vi "Flash LED.vi"(8 "Error In":errorcluster, 10 "Interval (S) (1 S)":dbl=1.0) -> (0 "Error Out":errorcluster, 2 "LED State":bool)   [LabVIEW 2016]
doc: "Toggles the USER LED on the cRIO at the specified when repetitively called.\nIt is designed to show genuine activity and will not cause the LED to Flash unless repetitively called\nat an interval shorter than the Interval. DR 11-10-2011"
uses:
  <vilib>/NI_Real-Time Target Support.lvlib
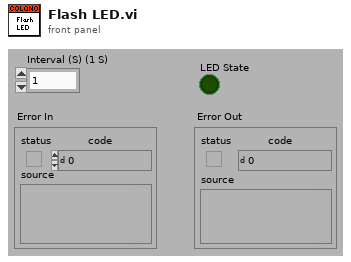
[diagram p1: front panel]
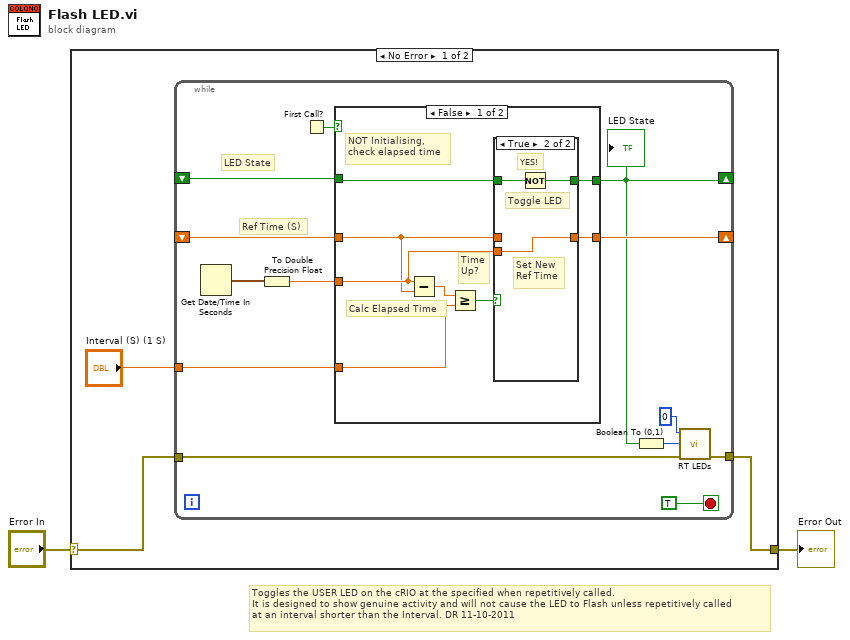
[diagram p0: block diagram]
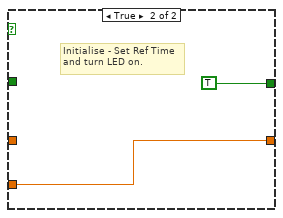
[diagram p3: hidden frame]
diagram:
  # "Toggles the USER LED on the cRIO at the specified when repetitively called.\nIt is designed to show genuine activity and will not cause the LED to Flash unless repetitively called\nat an interval shorter than the Interval. DR 11-10-2011"
  n1 = case shown="No Error" "Error In" {
    selector: "Error In" -> [w4 w34]
    tunnel: [w3 w34] -> w1
    frame No Error {
      n2 = while {
        shift-right: [w14] -> _
        shift-left: _ -> [w13]
        shift-right: [w6] -> _
        shift-left: _ -> [w12]
        tunnel: "Interval (S) (1 S)" -> [w11]
        tunnel: w4 -> [w10]
        tunnel: [w9] -> w3
        stop <- TRUE stop-if-true
        # "LED State"
        # "Ref Time (S)"
        n3 = Get Date/Time In Seconds() -> (seconds since 1Jan1904=w17:timestamp)
        n4 = To Double Precision Float(number=w17) -> (double precision float=w15:dbl)
        n5 = First Call?() -> (First Call?: T/F=w16:bool)
        n6 = case shown="False" w16 {
          tunnel: w15 -> [w23 w33]
          tunnel: [w22 w33] -> w14
          tunnel: w13 -> [w19 _]
          tunnel: [w21 TRUE ("LED")] -> w6
          tunnel: w11 -> [w25 _]
          tunnel: w12 -> [w20 _]
          frame False {
            # "NOT Initialising,\ncheck elapsed time"
            # "Time\nUp?"
            # "Calc Elapsed Time"
            n7 = Subtract(x=w23, y=w19) -> (x-y=w26:dbl)
            n8 = Greater Or Equal?(x=w26, y=w25) -> (x >= y?=w24:bool)
            n9 = case shown="True" w24 {
              tunnel: w23 -> [_ w31]
              tunnel: [w27 w31] -> w22
              tunnel: [w28 w30] -> w21
              tunnel: w20 -> [w28 w29]
              tunnel: w19 -> [w27 _]
              frame False {
                # "Keep same\nRef Time"
                # "NO!"
              }
              frame True {
                # "Toggle LED"
                # "YES!"
                # "Set New\nRef Time"
                n10 = Not(x=w29) -> (.not. x?=w30:bool)
              }
            }
          }
          frame True {
            # "Initialise - Set Ref Time\nand turn LED on."
          }
        }
        "LED State" <- w6
        n11 = Boolean To (0,1)(Boolean=w6) -> (0, 1=w7:i16)
        n12 = call <vilib>:"RT LEDs.vi"("error in (no error)"=w10, "State"=w7, "LED Num"=0) -> ("error out"=w9:errorcluster)  [unwired: 3 in, 1 out]
      }
    }
    frame Error {
    }
  }
  "Error Out" <- w1
